vi "CAN Enumerate.vi"(8 "error in (no error)":errorcluster) -> (0 "error out":errorcluster, 2 "Device Numbers":u8[](array[numeric]))   [LabVIEW 2009, in "CAN.lvlib"]
uses:
  CAN.lvlib
  SubVIs/CAN System Message IDs.ctl
panel:
  in  "error IO":errorcluster
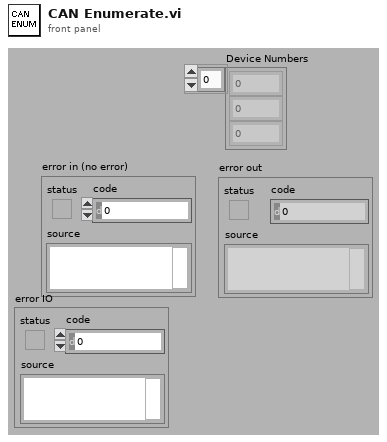
[diagram p1: front panel]
types:
  T1 = typedef "CAN.lvlib/CAN System Message IDs.ctl" = u32
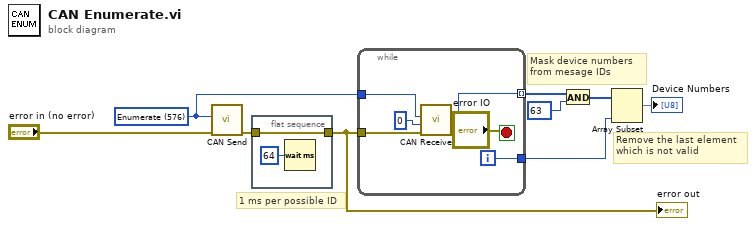
[diagram p0: block diagram]
diagram:
  w9 = T1 576 items=["Device Assignment"=128, "Device Query"=192, "Sync Update"=384, "Firmware Update"=448, "Firmware Version"=512, "Enumerate"=576] ("CAN System Message IDs")
  # "Remove the last element\nwhich is not valid"
  # "1 ms per possible ID"
  # "Mask device numbers\nfrom mesage IDs"
  n1 = call "CAN Send.vi"("error in (no error)"="error in (no error)", "messageID"=w9) -> ("error out"=w1:errorcluster)  [unwired: 1 in, 8 out]
  n2 = flat-sequence {
    tunnel: [w11] -> w2
    tunnel: w1 -> [w11]
    frame #0 {
      n3 = Wait (ms)(milliseconds to wait=u32 64) -> ()  [unwired: 1 out]
    }
  }
  n4 = while {
    tunnel: w2 -> [w17]
    tunnel: w9 -> [w16]
    tunnel: [w15] -> w8 mode=indexing
    tunnel: [w14] -> w5
    i -> [w14]
    stop <- "error IO" stop-if-true
    n5 = call "CAN Receive.vi"("error in (no error)"=w17, "timeoutMs"=u32 0, "Message ID"=w16) -> ("Message ID Out"=w15:u32)  [unwired: 8 out]
  }
  n6 = And(x=w8, y=u8 63 ("Message ID Out")) -> (x .and. y?=w6:u32[])
  n7 = Array Subset(array=w6, length=w5) -> (→"Device Numbers":u32[])  [unwired: 1 in]
  "error out" <- w2
